vi "Servo To Step.vi"(8 "Step Position":dbl, 10 "Rudder":dbl, 11 "Step":bool) -> (0 "Direction":bool, 1 "Step":bool, 3 "New Position":dbl)   [LabVIEW 2014]
panel:
  # "This subVI makes a stepper look like an RC/Servo\nIt compares curreny position to commanded position\nand outputs steps in teh right direction until the two are equal"
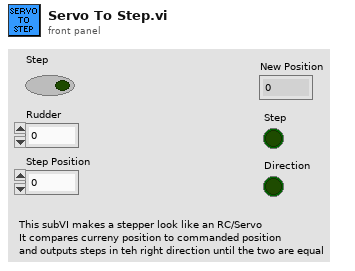
[diagram p1: front panel]
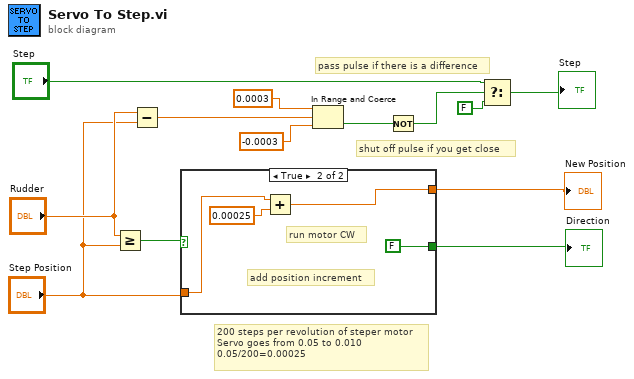
[diagram p0: block diagram]
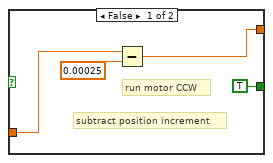
[diagram p2: hidden frame]
diagram:
  # "pass pulse if there is a difference"
  # "shut off pulse if you get close"
  # "200 steps per revolution of steper motor\nServo goes from 0.05 to 0.010\n0.05/200=0.00025"
  n1 = Greater Or Equal?(x="Rudder", y="Step Position") -> (x >= y?=w13:bool)
  n2 = Subtract(x="Rudder", y="Step Position") -> (x-y=w1:dbl)
  n3 = case shown="True" w13 {
    tunnel: [TRUE FALSE] -> w12
    tunnel: "Step Position" -> [w16 w18]
    tunnel: [w14 w20] -> w11
    frame False {
      # "subtract position increment"
      # "run motor CCW"
      n4 = Subtract(x=w16, y=0.00025) -> (x-y=w14:dbl)
    }
    frame True {
      # "add position increment"
      # "run motor CW"
      n5 = Add(x=w18, y=0.00025 ("x")) -> (x+y=w20:dbl)
    }
  }
  "Direction" <- w12
  "New Position" <- w11
  n6 = In Range and Coerce(upper limit=0.0003, x=w1, lower limit=-0.0003) -> (In Range?=w8:bool)  [unwired: 1 out]
  n7 = Not(x=w8) -> (.not. x?=w5:bool)
  n8 = Select(t="Step", s=w5, f=FALSE ("t")) -> (s? t:f=→"Step":bool)
